vi "Close Document.vi"(8 "error in (no error)":errorcluster, 11 "xwpfDocument in":refnum<class "xwpfDocument.lvclass">) -> (0 "error out":errorcluster, 3 "xwpfDocument out":refnum<class "xwpfDocument.lvclass">)   [LabVIEW 2017, in "Word_Specific.lvlib" / "xwpfDocument.lvclass"]
uses:
  xwpfDocument.lvclass
  xwpfDocument.lvclass/xwpfDocument.ctl
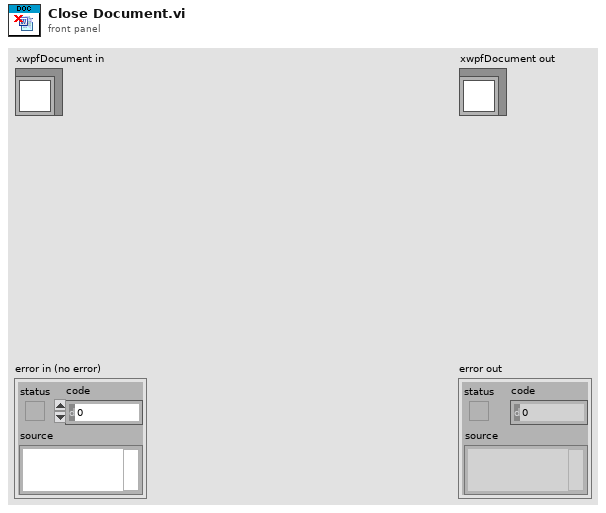
[diagram p1: front panel]
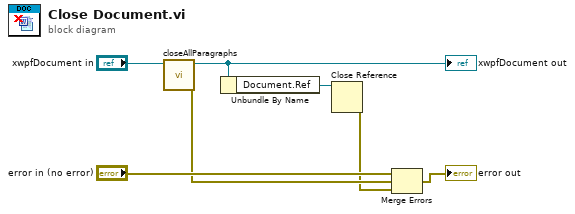
[diagram p0: block diagram]
diagram:
  n1 = call "closeAllParagraphs.vi"("xwpfDocument in"="xwpfDocument in") -> ("error out"=w2:errorcluster, "xwpfDocument out"=w5:refnum<class "xwpfDocument.lvclass">)  [unwired: 9 in]
  "xwpfDocument out" <- w5
  n2 = Unbundle By Name(w5) -> ("Document.Ref"=w4:refnum<k24>)
  n3 = Close Reference(reference=w4) -> (error out=w1:errorcluster)  [unwired: 1 in]
  n4 = Merge Errors("error in (no error)", w2, w1) -> (→"error out":errorcluster)
